vi "Get Module Path.vi"(8 "error in (no error)":errorcluster, 9 "Array 2":bool[](array[boolean]), 10 "Level":i32, 11 "path":path) -> (0 "error out":errorcluster, 1 "path out":path, 3 "Selected Path":path)   [LabVIEW 2025]
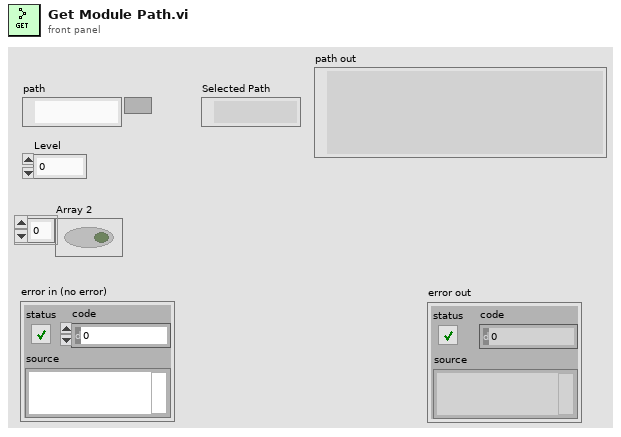
[diagram p1: front panel]
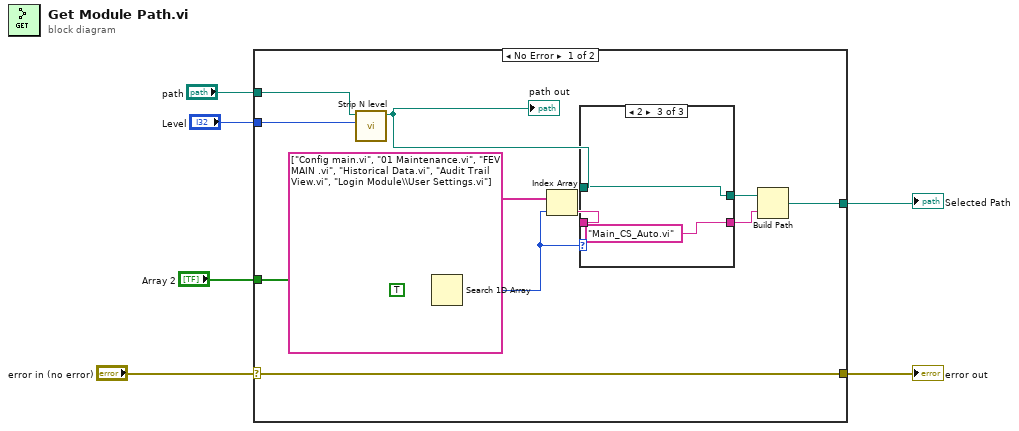
[diagram p0: block diagram]
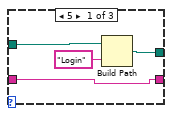
[diagram p2: hidden frame]
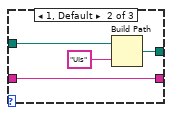
[diagram p3: hidden frame]
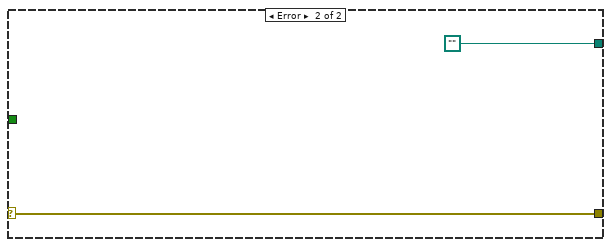
[diagram p4: hidden frame]
diagram:
  n1 = case shown="No Error" "error in (no error)" {
    selector: "error in (no error)" -> [w14 w30]
    tunnel: [w14 w30] -> w5
    tunnel: "path" -> [w13 _]
    tunnel: "Level" -> [w12 _]
    tunnel: [w11 path ""] -> w2
    tunnel: "Array 2" -> [w10 _]
    frame No Error {
      n2 = call "Strip N level.vi"("Level"=w12, "path in"=w13) -> ("path out"=w18:path)  [unwired: 9 in]
      "path out" <- w18
      n3 = Search 1D Array(1D array=w10, element=TRUE) -> (index of element=w9:i32)  [unwired: 1 in]
      n4 = Index Array(array=string[] ["Config main.vi", "01 Maintenance.vi", "FEV MAIN .vi", "Historical Data.vi", "Audit Trail View.vi", "Login Module\\User Settings.vi"], index=w9) -> (element=w8:string)
      n5 = case shown="2" w9 {
        tunnel: w18 -> [w22 w25 w27]
        tunnel: [w21 w24 w27] -> w17
        tunnel: w8 -> [w19 w23 _]
        tunnel: [w19 w23 "Main_CS_Auto.vi" ("name or relative path")] -> w7
        frame 5 {
          n6 = Build Path(base path=w22, name or relative path="Login") -> (appended path=w21:path)
        }
        frame 1, Default {
          n7 = Build Path(base path=w25, name or relative path="UIs") -> (appended path=w24:path)
        }
        frame 2 {
        }
      }
      n8 = Build Path(base path=w17, name or relative path=w7) -> (appended path=w11:path)
    }
    frame Error {
    }
  }
  "error out" <- w5
  "Selected Path" <- w2
